vi "get multiple lockin status.vi"(7 "Device channel names":string[](array[string]), 8 "error in (no error)":errorcluster, 11 "SRS830 addresses":refnum<visa-resource-name>[](array[refnum])) -> (0 "error out":errorcluster, 2 "Status output":string, 3 "SRS830 addresses out":refnum<visa-resource-name>[](array[refnum]))   [LabVIEW 2024]
panel:
  out "concatenated string":string
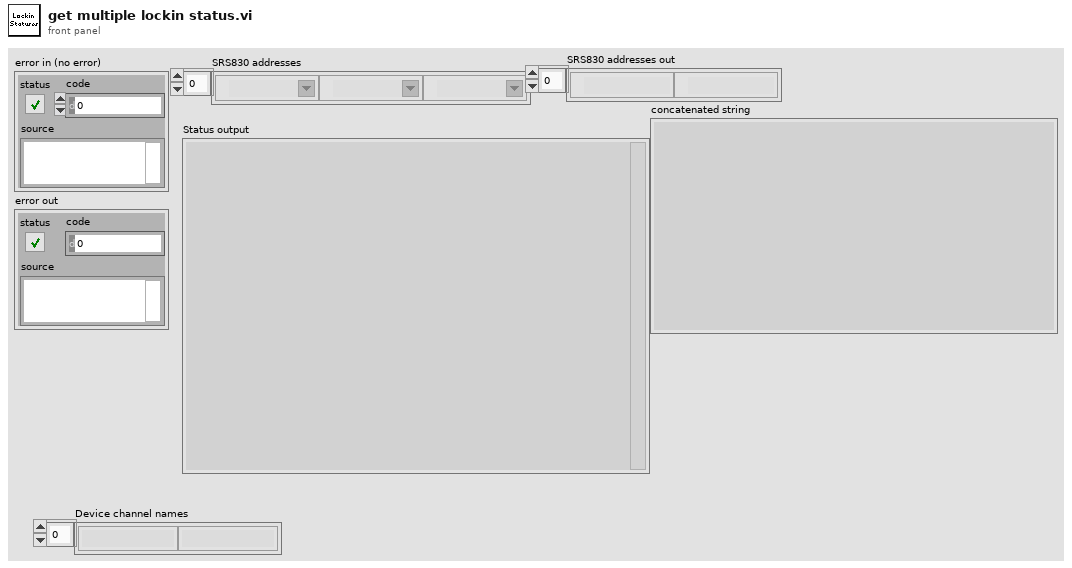
[diagram p1: front panel]
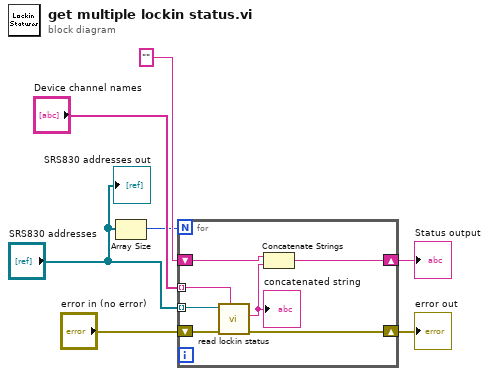
[diagram p0: block diagram]
diagram:
  n1 = Array Size(array="SRS830 addresses") -> (size(s)=w1:i32)
  n2 = for {
    N: w1 -> [_]
    tunnel: "SRS830 addresses" -> [w13] mode=indexing
    shift-right: [w12] -> w6
    shift-left: "error in (no error)" -> [w14]
    tunnel: "Device channel names" -> [w11] mode=indexing
    shift-right: [w9] -> w3
    shift-left: "" -> [w10]
    n3 = call "read lockin status.vi"("Device channel name"=w11, "error in (no error)"=w14, "SRS830 address"=w13) -> ("error out"=w12:errorcluster, "concatenated string"=w8:string)  [unwired: 6 in, 1 out]
    "concatenated string" <- w8
    n4 = Concatenate Strings(w10, w8) -> (w9:string)
  }
  "error out" <- w6
  "Status output" <- w3
  "SRS830 addresses out" <- "SRS830 addresses"
